vi "Pass State Machine.vi"   [LabVIEW 2013]
uses:
  typedefs/fg_typedef.ctl
  typedefs/subStates.ctl
types:
  T1 = typedef "subStates.ctl" = enum16{"null", "wait", "driver control", "auto", "manual override", "hold position", "rotate", "pickup", "pass", "load-shoot", "load-pass", "goto shoot", "shoot", "cancel", "end"}
  T2 = typedef "fg_typedef.ctl" = enum16{"Get", "Set"}
  T3 = typedef "WPI_DigitalInputDevRef.ctl" = cluster{"DevStatus":errorcluster, "DIO Channel":T4, "Digital Module":T5}
  T4 = typedef "FPGA_DIOChannel.ctl" = enum8{"DIO 1", "DIO 2", "DIO 3", "DIO 4", "DIO 5", "DIO 6", "DIO 7", "DIO 8", "DIO 9", "DIO 10", "DIO 11", "DIO 12", "DIO 13", "DIO 14", "Invalid"}
  T5 = typedef "FPGA_TypedefDigitalModule.ctl" = enum16{"Digital Module 1", "Digital Module 2"}
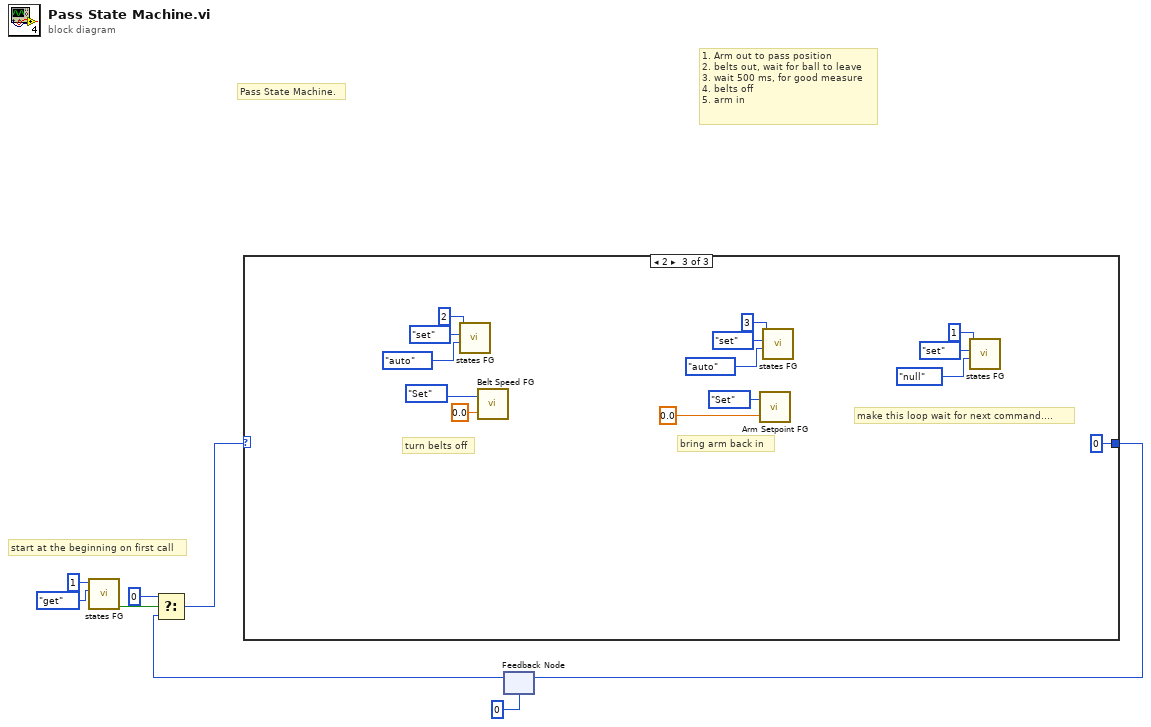
[diagram p0: block diagram]
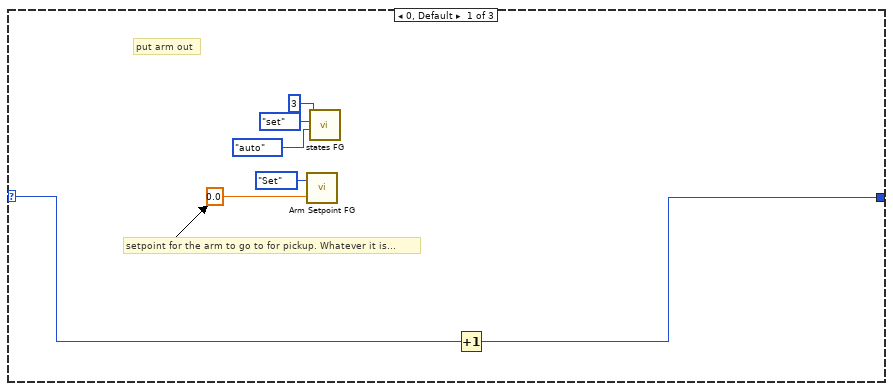
[diagram p2: hidden frame]
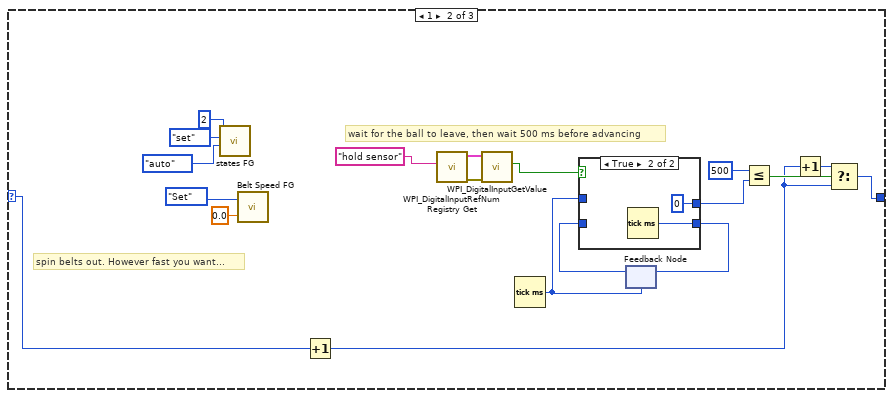
[diagram p3: hidden frame]
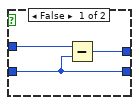
[diagram p4: hidden frame]
diagram:
  # "1. Arm out to pass position\n2. belts out, wait for ball to leave\n3. wait 500 ms, for good measure\n4. belts off\n5. arm in"
  # "Pass State Machine."
  # "start at the beginning on first call"
  n1 = call "states FG.vi"("menu (get)"=enum16{"set", "get"}."get", "Loop ID"=1) -> ("first call?"=w1:bool)  [unwired: 6 in, 3 out]
  n2 = feedback #1(0) -> (w4:i32)
  n3 = Select(t=0, s=w1, f=w4) -> (s? t:f=w3:i32)
  n4 = case shown="2" w3 {
    selector: w3 -> [w10 w34 _]
    tunnel: [w9 w16 0] -> w7
    frame 0, Default {
      # "setpoint for the arm to go to for pickup. Whatever it is..."
      # "put arm out"
      n5 = call "Arm Setpoint FG.vi"("Setpoint In"=0.0, "Menu"=fg_typedef."Set") -> ()  [unwired: 1 out]
      n6 = call "states FG.vi"("subState in"=subStates."auto", "menu (get)"=enum16{"set", "get"}."set", "Loop ID"=3) -> ()  [unwired: 5 in, 4 out]
      n7 = Increment(x=w10) -> (x+1=w9:i32)
    }
    frame 1 {
      # "wait for the ball to leave, then wait 500 ms before advancing"
      # "spin belts out. However fast you want..."
      n8 = call "states FG.vi"("subState in"=subStates."auto", "menu (get)"=enum16{"set", "get"}."set", "Loop ID"=2) -> ()  [unwired: 5 in, 4 out]
      n9 = call "Belt Speed FG.vi"("Speed In"=0.0, "Menu"=fg_typedef."Set") -> ()  [unwired: 1 out]
      n10 = Increment(x=w34) -> (x+1=w18:i32)
      n11 = call <vilib>:"WPI_DigitalInputRefNum Registry Get.vi"("refnum name"="hold sensor") -> ("error out"=w27:errorcluster, "DigitalInputDevRef"=w26:T3)  [unwired: 9 in]
      n12 = call <vilib>:"WPI_DigitalInputGetValue.vi"("error in (no error)"=w27, "DigitalInputDevRef"=w26) -> ("Value"=w20:bool)  [unwired: 7 in, 2 out]
      n13 = Tick Count (ms)() -> (millisecond timer value=w22:u32)
      n14 = feedback #2(w22) -> (w21:u32)
      n15 = case shown="True" w20 {
        tunnel: [w37 w39] -> w25
        tunnel: w21 -> [w37 _]
        tunnel: [w36 u32 0] -> w24
        tunnel: w22 -> [w35 _]
        frame False {
          n16 = Subtract(x=w35, y=w37) -> (x-y=w36:u32)
        }
        frame True {
          n17 = Tick Count (ms)() -> (millisecond timer value=w39:u32)
        }
      }
      n18 = feedback-in #2(w25) -> ()
      n19 = Less Or Equal?(x=u32 500, y=w24) -> (x <= y?=w19:bool)
      n20 = Increment(x=w18) -> (x+1=w17:i32)
      n21 = Select(t=w17, s=w19, f=w18) -> (s? t:f=w16:i32)
    }
    frame 2 {
      # "make this loop wait for next command...."
      # "bring arm back in"
      # "turn belts off"
      n22 = call "states FG.vi"("subState in"=subStates."auto", "menu (get)"=enum16{"set", "get"}."set", "Loop ID"=2) -> ()  [unwired: 5 in, 4 out]
      n23 = call "Belt Speed FG.vi"("Speed In"=0.0, "Menu"=fg_typedef."Set") -> ()  [unwired: 1 out]
      n24 = call "Arm Setpoint FG.vi"("Setpoint In"=0.0, "Menu"=fg_typedef."Set") -> ()  [unwired: 1 out]
      n25 = call "states FG.vi"("subState in"=subStates."auto", "menu (get)"=enum16{"set", "get"}."set", "Loop ID"=3) -> ()  [unwired: 5 in, 4 out]
      n26 = call "states FG.vi"("subState in"=subStates."null", "menu (get)"=enum16{"set", "get"}."set", "Loop ID"=1) -> ()  [unwired: 5 in, 4 out]
    }
  }
  n27 = feedback-in #1(w7) -> ()
